vi "SendGetAnalogCommand.vi"(3 "Pin":u8=1 max=11, 4 "Port Destination":u16, 5 "Adresse IP Destination":u32, 6 "entrée d'erreur":errorcluster caption="entrée d'erreur (pas d'erreur)", 7 "Connexion réseau UDP en entrée":refnum<k16>) -> (0 "sortie d'erreur 2":errorcluster caption="sortie d'erreur", 1 "Connexion réseau UDP en sortie":refnum<k16>)   [LabVIEW 2021]
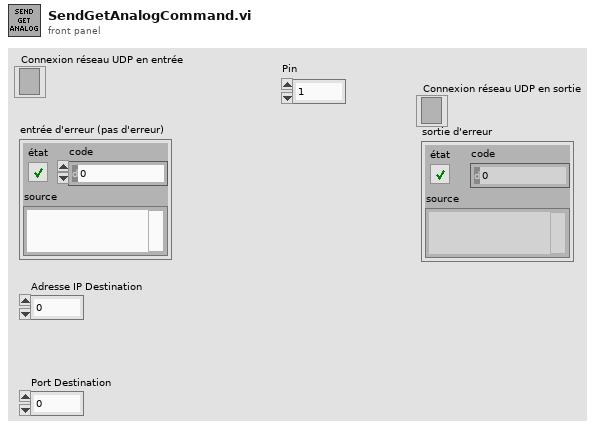
[diagram p1: front panel]
types:
  T1 = typedef "CommandType.ctl" = u8[]
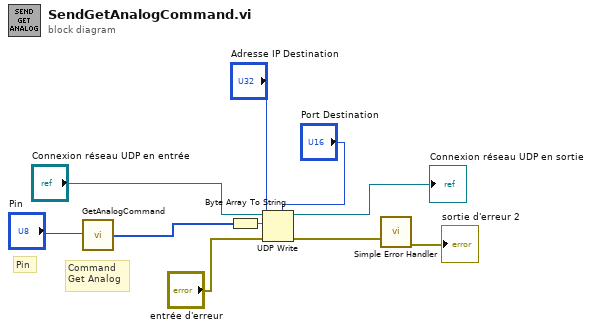
[diagram p0: block diagram]
diagram:
  # "Command \nGet Analog"
  # "Pin"
  n1 = call "GetAnalogCommand.vi"("Pin"="Pin") -> ("Command"=w5:T1)
  n2 = Byte Array To String(unsigned byte array=w5) -> (string=w6:string)
  n3 = UDP Write(address="Adresse IP Destination", port or service name="Port Destination", connection ID="Connexion réseau UDP en entrée", data in=w6, 8:"entrée d'erreur") -> (error out=w1:errorcluster, 3:→"Connexion réseau UDP en sortie":refnum<k16>)  [unwired: 1 in]
  n4 = call <vilib>:"Simple Error Handler.vi"("error in (no error)"=w1) -> ("error out"=→"sortie d'erreur 2":errorcluster)  [unwired: 4 in, 4 out]
